vi "BRig_dataBlock_nTrial_rebiasing.vi"() -> (2 "output_nTrial_rebiasing":i32)   [LabVIEW 2014]
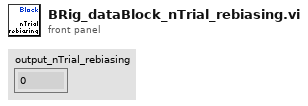
[diagram p1: front panel]
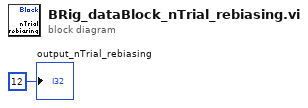
[diagram p0: block diagram]
diagram:
  "output_nTrial_rebiasing" <- 12 ("output_iBlock")
